vi "User Event Abort.vi"(7 "Action":T1, 8 "Error In":errorcluster) -> (0 "Error Out":errorcluster, 3 "User Event Out":refnum<user-event>)   [LabVIEW 2019]
uses:
  Controls/UE Abort Action.ctl
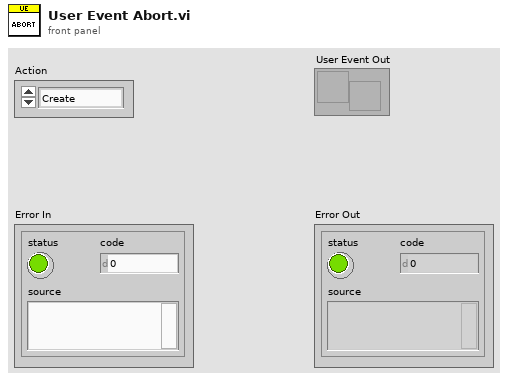
[diagram p1: front panel]
types:
  T1 = typedef "UE Abort Action.ctl" = enum16{"Create", "Get", "Destroy"}
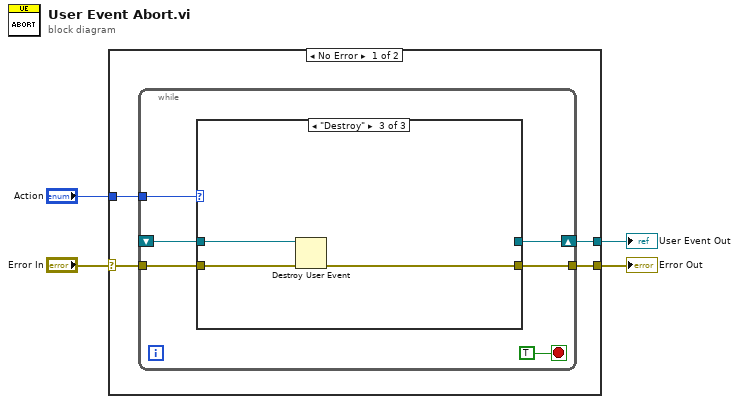
[diagram p0: block diagram]
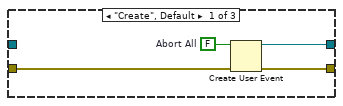
[diagram p2: hidden frame]
diagram:
  n1 = case shown="No Error" "Error In" {
    selector: "Error In" -> [w7 w24]
    tunnel: [w6 w24] -> w3
    tunnel: "Action" -> [w8 _]
    tunnel: [w5 _] -> w1
    frame No Error {
      n2 = while {
        tunnel: w8 -> [w14]
        tunnel: w7 -> [w13]
        tunnel: [w12] -> w6
        shift-right: [w11] -> w5
        shift-left: _ -> [w10]
        stop <- TRUE stop-if-true
        n3 = case shown="\"Destroy\"" w14 {
          tunnel: w13 -> [w18 w19 w23]
          tunnel: [w17 w19 w21] -> w12
          tunnel: [w16 w20 _] -> w11
          tunnel: w10 -> [_ w20 w22]
          frame "Create", Default {
            w15 = FALSE  # Abort All
            n4 = Create User Event(user event datatype=w15, error in=w18) -> (user event=w16:refnum<user-event>, error out=w17:errorcluster)
          }
          frame "Get" {
          }
          frame "Destroy" {
            n5 = Destroy User Event(user event=w22, error in=w23) -> (error out=w21:errorcluster)
          }
        }
      }
    }
    frame Error {
    }
  }
  "Error Out" <- w3
  "User Event Out" <- w1
